vi "PRUEBAS.vi"() -> ()   [LabVIEW 2019]
uses:
  controls/M1states.ctl
  <vilib>/NI/Modbus Library/API/Wrapper/Create TCP Master.vi
  <vilib>/NI/Modbus Library/API/Master/Modbus Master.lvclass
  <vilib>/NI/Modbus Library/API/Wrapper/API Main.lvlib
panel:
  in  "open":bool
  in  "close":bool
  out "Tank":dbl(slide) scale=0.0..10.0
  out "register values":u16[](array[numeric])
  out "error out":errorcluster
  in  "Stop":bool
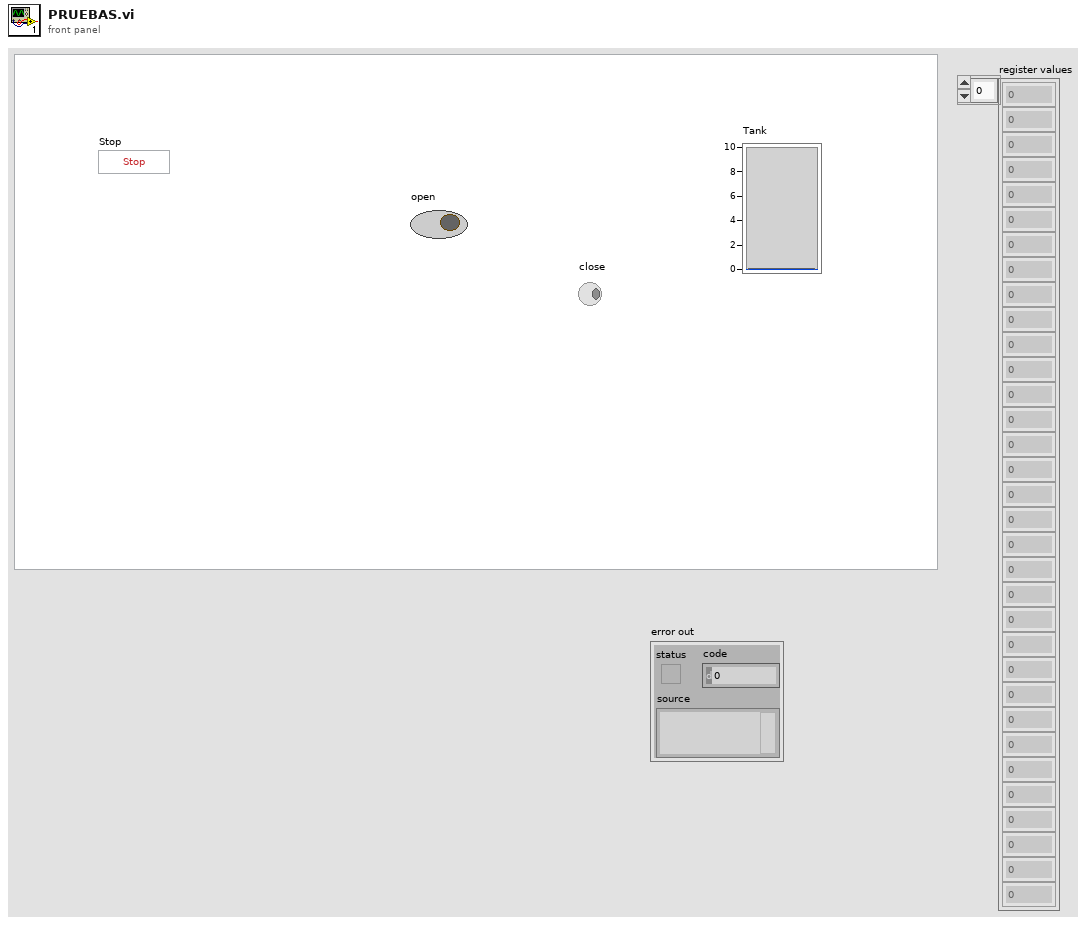
[diagram p1: front panel]
types:
  T1 = typedef "M1states.ctl" = enum16{"VERIFICACION", "HERVIR", "REPOSO", "LAVADO"}
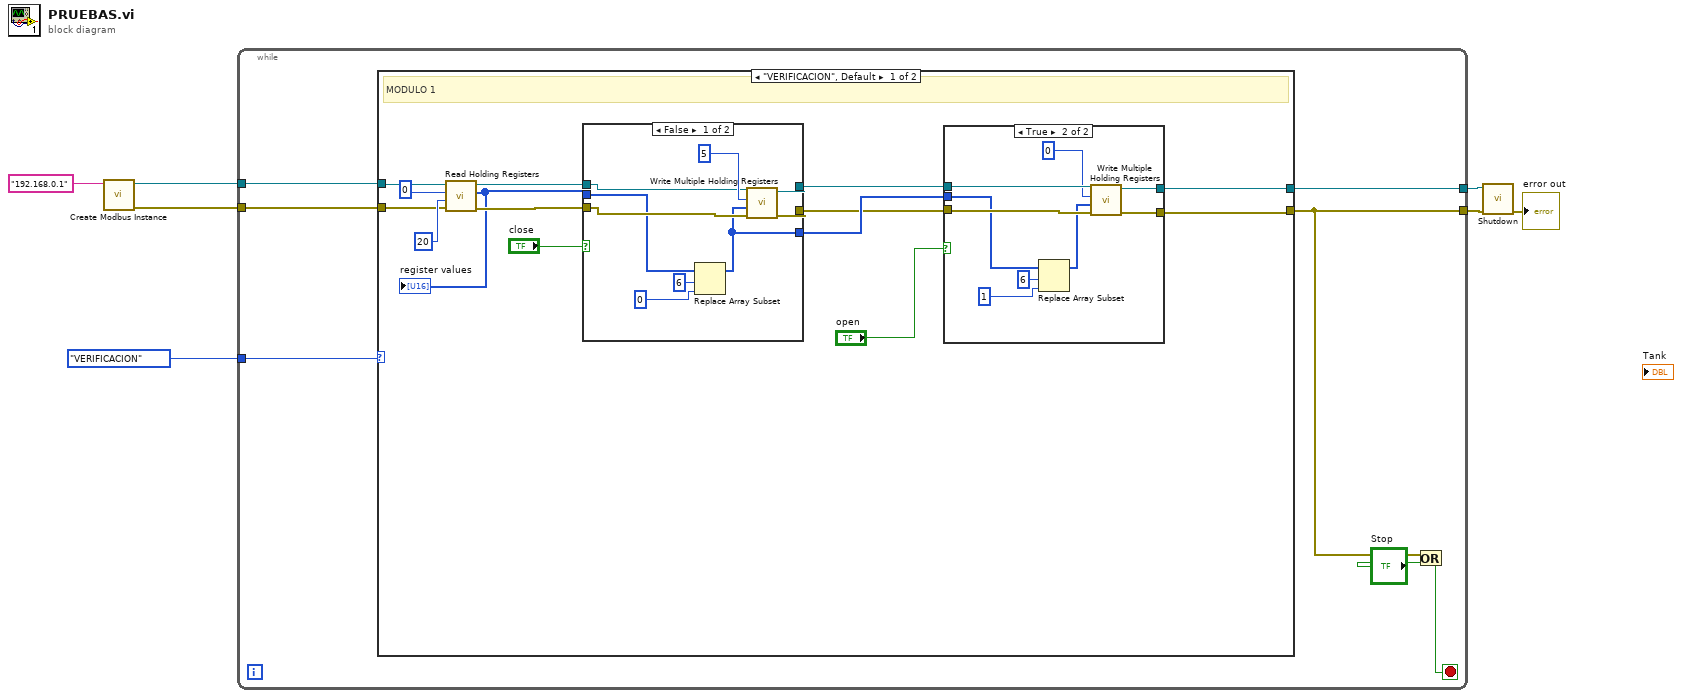
[diagram p0: block diagram]
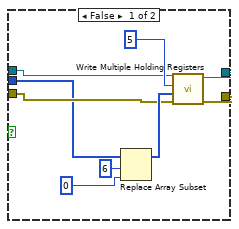
[diagram p2: hidden frame]
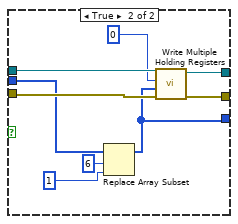
[diagram p3: hidden frame]
diagram:
  n1 = call-poly <vilib>:"Create Modbus Instance.vi"("address"="192.168.0.1") -> ("error out"=w6:errorcluster, "TCP master instance"=w7:refnum<class "Modbus Master.lvclass">)  [unwired: 9 in]
  n2 = while {
    tunnel: w7 -> [w11]
    tunnel: w6 -> [w12]
    tunnel: [w10] -> w4
    tunnel: [w9] -> w5
    tunnel: M1states."VERIFICACION" -> [w8]
    stop <- w13 stop-if-true
    n3 = case shown="\"VERIFICACION\", Default" w8 {
      tunnel: w12 -> [w22 w65]
      tunnel: w11 -> [w23 w66]
      tunnel: [w17 w66] -> w10
      tunnel: [w16 w65] -> w9
      frame "VERIFICACION", Default {
        # "MODULO 1"
        n4 = call-dynamic "Read Holding Registers.vi"("error in"=w22, "number of inputs"=u16 20, "starting address"=u16 0, "Modbus master in"=w23) -> ("error out"=w25:errorcluster, "register values"=w24:u16[], "Modbus master out"=w26:refnum<class "Modbus Master.lvclass">)  [unwired: 5 in]
        "register values" <- w24
        n5 = case shown="False" "close" {
          tunnel: w26 -> [w52 w64]
          tunnel: [w49 w63] -> w19
          tunnel: w25 -> [w51 w62]
          tunnel: [w48 w61] -> w18
          tunnel: w24 -> [w50 w59]
          tunnel: [w47 w56] -> w20
          frame False {
            n6 = Replace Array Subset(array=w50, new element=u16 0, index=6) -> (w47:u16[])
            n7 = call-dynamic "Write Multiple Holding Registers.vi"("error in"=w51, "registers to write"=w47, "starting address"=u16 5, "Modbus master in"=w52) -> ("error out"=w48:errorcluster, "Modbus master out"=w49:refnum<class "Modbus Master.lvclass">)  [unwired: 6 in]
          }
          frame True {
            n8 = Replace Array Subset(array=w59, new element=u16 1, index=6) -> (w56:u16[])
            n9 = call-dynamic "Write Multiple Holding Registers.vi"("error in"=w62, "registers to write"=w56, "starting address"=u16 0, "Modbus master in"=w64) -> ("error out"=w61:errorcluster, "Modbus master out"=w63:refnum<class "Modbus Master.lvclass">)  [unwired: 6 in]
          }
        }
        n10 = case shown="True" "open" {
          tunnel: w19 -> [w33 w46]
          tunnel: [w30 w45] -> w17
          tunnel: w18 -> [w32 w44]
          tunnel: [w29 w43] -> w16
          tunnel: w20 -> [w31 w41]
          frame False {
            n11 = Replace Array Subset(array=w31, new element=u16 0, index=6) -> (w36:u16[])
            n12 = call-dynamic "Write Multiple Holding Registers.vi"("error in"=w32, "registers to write"=w36, "starting address"=u16 5, "Modbus master in"=w33) -> ("error out"=w29:errorcluster, "Modbus master out"=w30:refnum<class "Modbus Master.lvclass">)  [unwired: 6 in]
          }
          frame True {
            n13 = Replace Array Subset(array=w41, new element=u16 1, index=6) -> (w40:u16[])
            n14 = call-dynamic "Write Multiple Holding Registers.vi"("error in"=w44, "registers to write"=w40, "starting address"=u16 0, "Modbus master in"=w46) -> ("error out"=w43:errorcluster, "Modbus master out"=w45:refnum<class "Modbus Master.lvclass">)  [unwired: 6 in]
          }
        }
      }
      frame "HERVIR" {
        # "MODULO 1"
      }
    }
    n15 = Or(x=w9, y="Stop") -> (x .or. y?=w13:bool)
  }
  n16 = call-dynamic "Shutdown.vi"("error in"=w5, "Modbus master in"=w4) -> ("error out"=→"error out":errorcluster)  [unwired: 9 in]
